vi "high_speed_digitizer_ao.vi"() -> ()   [LabVIEW 2014]
uses:
  <vilib>/Utility/error.llb/DialogType.ctl
  <vilib>/addons/h5labview2/file/H5Fmode.ctl
  <vilib>/DAQmx/create/channels.llb/DAQmx Create Channel (AI-Voltage-Basic).vi
  <vilib>/DAQmx/configure/timing.llb/DAQmx Timing (Sample Clock).vi
  <vilib>/DAQmx/create/channels.llb/DAQmx Create Channel (AO-Voltage-Basic).vi
  <vilib>/DAQmx/configure/trigger.llb/DAQmx Start Trigger (Digital Edge).vi
  <vilib>/DAQmx/configure/trigger.llb/DAQmx Start Trigger (Analog Edge).vi
  <vilib>/DAQmx/configure/trigger.llb/DAQmx Reference Trigger (Digital Edge).vi
  <vilib>/DAQmx/configure/trigger.llb/DAQmx Reference Trigger (Analog Edge).vi
  <vilib>/DAQmx/read.llb/DAQmx Read (Analog 2D DBL NChan NSamp).vi
  <vilib>/DAQmx/write.llb/DAQmx Write (Analog Wfm 1Chan NSamp).vi
  <vilib>/addons/h5labview2/base/lib_path.vi
  <vilib>/addons/h5labview2/base/H5Equery.vi
  <vilib>/addons/h5labview2/dataset/H5Dwrite.llb/H5Dwrite.xnode
  <vilib>/addons/h5labview2/attrib/H5Awrite.llb/H5Awrite.xnode
  <vilib>/addons/h5labview2/base/hid_t.ctl
  <resource>/objmgr/daqmx.rc
  <vilib>/addons/h5labview2/file/H5F.lvlib
  <vilib>/addons/h5labview2/group/H5G.lvlib
  National Instruments Downloads/LabVIEW FPGA English/FPGA Timekeeper 1.1b0/FPGA Timekeeper.lvlib
  <vilib>/measure/NI_MABase.lvlib
panel:
  in  "proc_amp_increment":dbl
  in  "proc_amp":dbl format="%0.2p"
  in  "synth_settle_time":u32
  in  "drive frequency increment":dbl
  in  "init drive frequency":dbl format="%0.2p"
  in  "drive amp increment":dbl
  in  "init drive amp":dbl format="%0.5p"
  in  "dc increment":dbl
  in  "init offset":dbl format="%0.2p"
  in  "Max Voltage 2":dbl=5.0
  in  "Min Voltage 2":dbl=-5.0
  in  "Physical Channel(s)":tag="Dev1/ao0"
  out "P_baratron [mbar]":dbl format="%#_3g"
  out "P_pirani [torr]":dbl format="%#_3g"
  out "P_cc [torr]":dbl format="%#_3g"
  out "T_elec_rack [C]":dbl
  out "T_opt_table [C]":dbl
  in  "Read pressures?":bool=TRUE
  in  "Read temps?":bool=TRUE
  in  "Num files":i32
  in  "File base name":string
  in  "Directory path":path
  out "Waveform Graph":dbl[][](graph)
  in  "Number of Samples":i32=500000
  in  "Trigger Type":T1(tab)=enum."Digital Start"
  in  "Edge":i32(ring)=10280 items=["Rising"=10280, "Falling"=10171]
  in  "Digital Trigger Source":tag="/Dev2/PFI0"
  in  "Level (V)":dbl format="%0.2f"
  in  "Hysteresis (V)":dbl
  in  "Slope":i32(ring)=10280 items=["Rising"=10280, "Falling"=10171]
  in  "Analog Trigger Source":string="APFI0"
  in  "Digital Ref Trigger Source":tag
  in  "Edge 2":i32(ring)=10280 items=["Rising"=10280, "Falling"=10171]
  in  "Pre-Trigger Samples":u32
  in  "Analog Ref Trigger Source":string="APFI0"
  in  "Slope 2":i32(ring)=10280 items=["Rising"=10280, "Falling"=10171]
  in  "Level (V) 2":dbl format="%0.2f"
  in  "Pre-Trigger Samples 2":u32
  in  "Sample Rate":dbl=300000.0
  in  "Sample Clock Source":tag="OnboardClock"
  in  "Terminal Configuration":i32(ring)=-1 items=["default"=-1, "RSE"=10083, "NRSE"=10078, "Differential"=10106, "Pseudodifferential"=12529]
  in  "Max Voltage":dbl=5.0
  in  "Min Voltage":dbl=-5.0
  in  "Physical Channel":tag="Dev2/ai0:2"
  out "Actual Sample Rate":dbl=1000.0 format="%0.2f"
  # "To configure and use a start trigger you must have the necessary tab selected above.  Not all hardware supports triggering--refer to your device documentation for more info."
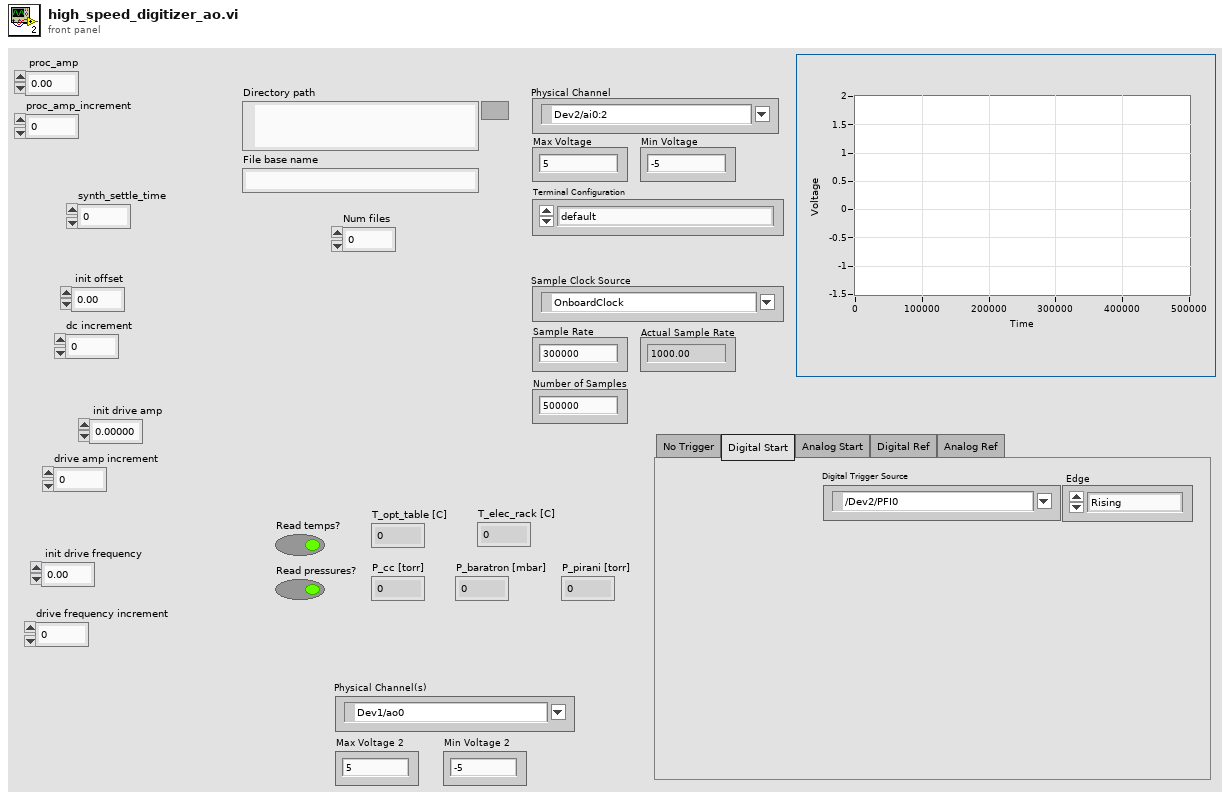
[diagram p1: front panel]
types:
  T1 = enum32{"No Trigger", "Digital Start", "Analog Start", "Digital Ref", "Analog Ref"}
  T2 = enum16{"Sine Wave", "Triangle Wave", "Square Wave", "Sawtooth Wave"}
  T3 = typedef "H5F.lvlib/H5Fmode.ctl" = enum16{"read-only", "read-write", "overwrite", "create new", "open or create"}
  T4 = typedef "DialogType.ctl" = u16
  T5 = typedef "hid_t.ctl" = i32
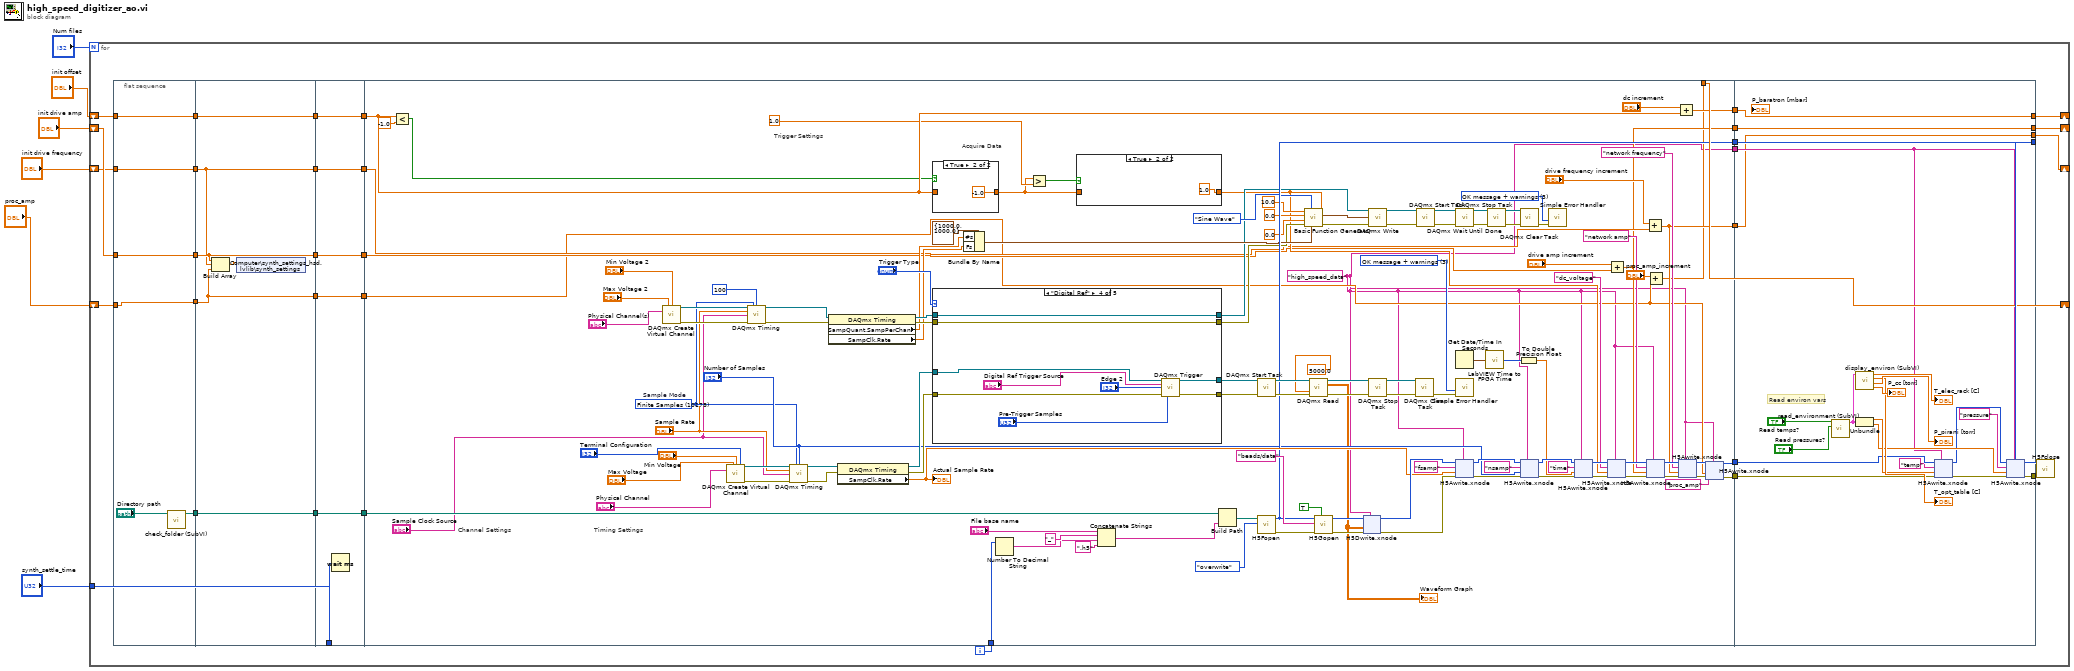
[diagram p0: block diagram]
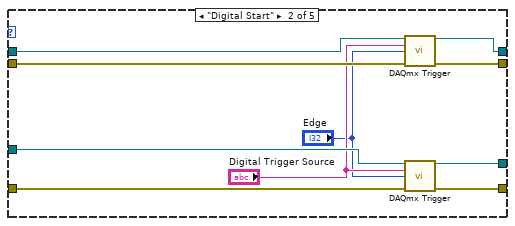
[diagram p5: hidden frame]
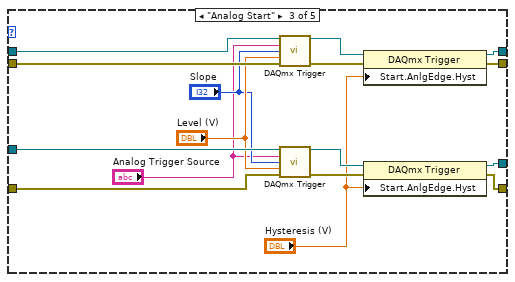
[diagram p6: hidden frame]
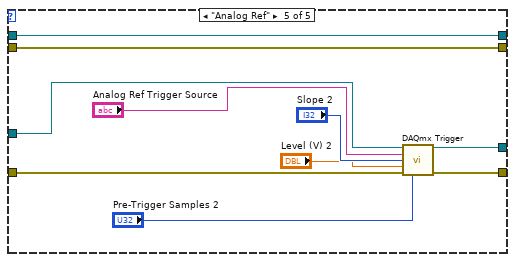
[diagram p7: hidden frame]
diagram:
  n1 = for {
    N: "Num files" -> [_]
    shift-right: [w32] -> _
    shift-left: "init offset" -> [w31]
    shift-right: [w20] -> _
    shift-left: "init drive amp" -> [w23]
    shift-right: [w13] -> _
    shift-left: "init drive frequency" -> [w18]
    tunnel: "synth_settle_time" -> [w12]
    shift-right: [w7] -> _
    shift-left: "proc_amp" -> [w10]
    i -> [w40]
    n2 = flat-sequence {
      tunnel: [w45] -> w30
      tunnel: [w44] -> w29
      tunnel: w31 -> [w44]
      tunnel: [w43] -> w24
      tunnel: w23 -> [w43]
      tunnel: w18 -> [w42]
      tunnel: [w42] -> w15
      tunnel: [w41] -> w11
      tunnel: w10 -> [w41]
      tunnel: w30 -> [w52]
      tunnel: [w52] -> w28
      tunnel: w29 -> [w51]
      tunnel: [w51] -> w26
      tunnel: w24 -> [w50]
      tunnel: [w50] -> w22
      tunnel: [w49] -> w16
      tunnel: w15 -> [w49]
      tunnel: w11 -> [w47]
      tunnel: [w47] -> w8
      tunnel: w28 -> [w58]
      tunnel: [w58] -> w27
      tunnel: w26 -> [w57]
      tunnel: [w57] -> w25
      tunnel: w22 -> [w56]
      tunnel: [w56] -> w21
      tunnel: [w55] -> w17
      tunnel: w16 -> [w55]
      tunnel: w12 -> [w54]
      tunnel: [w53] -> w9
      tunnel: w8 -> [w53]
      tunnel: w40 -> [w157]
      tunnel: [w137] -> w37
      tunnel: [w66] -> w36
      tunnel: [w64] -> w35
      tunnel: [w61] -> w34
      tunnel: w27 -> [w130]
      tunnel: w25 -> [w95]
      tunnel: [w92] -> w33
      tunnel: w21 -> [w80]
      tunnel: [w71] -> w19
      tunnel: w17 -> [w78]
      tunnel: [w70] -> w14
      tunnel: w9 -> [w63]
      tunnel: [w68] -> w7
      tunnel: [w386] -> w38
      tunnel: [w396] -> w39
      tunnel: w37 -> [w396]
      tunnel: w36 -> [w388]
      tunnel: w35 -> [w383]
      tunnel: w34 -> [w381]
      tunnel: [w378] -> w32
      tunnel: w33 -> [w378]
      tunnel: [w377] -> w20
      tunnel: w19 -> [w377]
      tunnel: [w376] -> w13
      tunnel: w14 -> [w376]
      frame #0 {
        n3 = call "check_folder (SubVI).vi"("path in"="Directory path") -> ("path out"=w45:path)  [unwired: 10 in]
      }
      frame #1 {
        n4 = Build Array(w50, w49, w47) -> (w48:dbl[])
        n5 = shared-variable "My Computer\\synth_settings_hsd.lvlib\\synth_settings"(w48) -> ()  [unwired: 1 in, 1 out]
      }
      frame #2 {
        n6 = Wait (ms)(milliseconds to wait=w54) -> ()  [unwired: 1 out]
      }
      frame #3 {
        w106 = T4 3 items=["no dialog", "OK message", "continue or stop message", "OK message + warnings", "continue/stop + warnings"] ("type of dialog (OK msg:1)")
        w61 = "high_speed_data" ("dataset name")
        w160 = T4 3 items=["no dialog", "OK message", "continue or stop message", "OK message + warnings", "continue/stop + warnings"] ("type of dialog (OK msg:1)")
        w99 = 10178 items=["Finite Samples"=10178, "Continuous Samples"=10123, "Hardware Timed Single Point"=12522]  # Sample Mode
        # "Acquire Data"
        # "Trigger Settings"
        # "Timing Settings"
        # "Channel Settings"
        n7 = Less?(x=w95, y=-1.0) -> (x < y?=w93:bool)
        n8 = call-poly <vilib>:"DAQmx Create Virtual Channel.vi"("maximum value"="Max Voltage 2", "minimum value"="Min Voltage 2", "physical channels"="Physical Channel(s)") -> ("task out"=w126:refnum<k21>, "error out"=w127:errorcluster)  [unwired: 11 in]
        n9 = call-poly <vilib>:"DAQmx Create Virtual Channel.vi"("maximum value"="Max Voltage", "minimum value"="Min Voltage", "input terminal configuration"="Terminal Configuration", "physical channels"="Physical Channel") -> ("task out"=w175:refnum<k21>, "error out"=w176:errorcluster)  [unwired: 10 in]
        n10 = call-poly <vilib>:"DAQmx Timing.vi"("task/channels in"=w126, "sample mode"=w99, "samples per channel"=100, "rate"="Sample Rate", "source"="Sample Clock Source", "error in"=w127) -> ("task out"=w129:refnum<k21>, "error out"=w128:errorcluster)  [unwired: 8 in]
        n11 = call-poly <vilib>:"DAQmx Timing.vi"("task/channels in"=w175, "sample mode"=w99, "samples per channel"="Number of Samples", "rate"="Sample Rate", "source"="Sample Clock Source", "error in"=w176) -> ("task out"=w178:refnum<k21>, "error out"=w177:errorcluster)  [unwired: 8 in]
        n12 = property class="DAQmx Timing"(reference=w129, error in=w128) -> (reference out=w122:refnum<k21>, error out=w121:errorcluster, "SampQuant.SampPerChan"=w119:dbl, "SampClk.Rate"=w118:dbl)
        n13 = property class="DAQmx Timing"(reference=w178, error in=w177) -> (reference out=w158:refnum<k21>, error out=w159:errorcluster, "SampClk.Rate"=w139:dbl)
        "Actual Sample Rate" <- w139
        n14 = case shown="True" w93 {
          tunnel: w95 -> [w235 _]
          tunnel: [w235 -1.0 ("offset")] -> w89
          frame False {
          }
          frame True {
          }
        }
        n15 = case shown="\"Digital Ref\"" "Trigger Type" {
          tunnel: w158 -> [w330 w340 w356 w365 w375]
          tunnel: w159 -> [w329 w339 w355 w364 w374]
          tunnel: [w330 w338 w354 w363 w369] -> w174
          tunnel: [w329 w337 w353 w362 w370] -> w173
          tunnel: w122 -> [w328 w336 w348 w358 w367]
          tunnel: w121 -> [w327 w335 w347 w357 w366]
          tunnel: [w328 w334 w346 w358 w367] -> w111
          tunnel: [w327 w333 w345 w357 w366] -> w113
          frame "No Trigger", Default {
          }
          frame "Digital Start" {
            n16 = call-poly <vilib>:"DAQmx Trigger.vi"("task/channels in"=w336, "source"="Digital Trigger Source", "edge"="Edge", "error in"=w335) -> ("task out"=w334:refnum<k21>, "error out"=w333:errorcluster)  [unwired: 10 in]
            n17 = call-poly <vilib>:"DAQmx Trigger.vi"("task/channels in"=w340, "source"="Digital Trigger Source", "edge"="Edge", "error in"=w339) -> ("task out"=w338:refnum<k21>, "error out"=w337:errorcluster)  [unwired: 10 in]
          }
          frame "Analog Start" {
            n18 = call-poly <vilib>:"DAQmx Trigger.vi"("task/channels in"=w348, "source"="Analog Trigger Source", "slope"="Slope", "level"="Level (V)", "error in"=w347) -> ("task out"=w350:refnum<k21>, "error out"=w349:errorcluster)  [unwired: 9 in]
            n19 = call-poly <vilib>:"DAQmx Trigger.vi"("task/channels in"=w356, "source"="Analog Trigger Source", "slope"="Slope", "level"="Level (V)", "error in"=w355) -> ("task out"=w352:refnum<k21>, "error out"=w351:errorcluster)  [unwired: 9 in]
            n20 = property class="DAQmx Trigger"(reference=w350, error in=w349, "Start.AnlgEdge.Hyst"="Hysteresis (V)") -> (reference out=w346:refnum<k21>, error out=w345:errorcluster)
            n21 = property class="DAQmx Trigger"(reference=w352, error in=w351, "Start.AnlgEdge.Hyst"="Hysteresis (V)") -> (reference out=w354:refnum<k21>, error out=w353:errorcluster)
          }
          frame "Digital Ref" {
            n22 = call-poly <vilib>:"DAQmx Trigger.vi"("task/channels in"=w365, "source"="Digital Ref Trigger Source", "edge"="Edge 2", "error in"=w364, "pretrigger samples per channel"="Pre-Trigger Samples") -> ("task out"=w363:refnum<k21>, "error out"=w362:errorcluster)  [unwired: 9 in]
          }
          frame "Analog Ref" {
            n23 = call-poly <vilib>:"DAQmx Trigger.vi"("task/channels in"=w375, "source"="Analog Ref Trigger Source", "slope"="Slope 2", "level"="Level (V) 2", "error in"=w374, "pretrigger samples per channel"="Pre-Trigger Samples 2") -> ("task out"=w369:refnum<k21>, "error out"=w370:errorcluster)  [unwired: 8 in]
          }
        }
        n24 = Bundle By Name(cluster=cluster{"Fs":dbl, "#s":dbl} {"Fs"=1000.0, "#s"=1000.0} ("sampling info"), "#s"=w119, "Fs"=w118) -> (w117:cluster{"Fs":dbl, "#s":dbl})
        n25 = Number To Decimal String(number=w157) -> (decimal integer string=w155:string)  [unwired: 1 in]
        n26 = Greater?(x=w89, y=1.0) -> (0:w90:bool)
        n27 = case shown="True" w90 {
          tunnel: w89 -> [w233 _]
          tunnel: [w233 1.0 ("offset")] -> w87
          frame False {
          }
          frame True {
          }
        }
        n28 = Concatenate Strings("File base name", "_", w155, ".h5") -> (w152:string)
        n29 = Build Path(base path=w130, name or relative path=w152) -> (appended path=w150:path)
        n30 = call <vilib>:"DAQmx Start Task.vi"("task/channels in"=w174, "error in"=w173) -> ("task out"=w172:refnum<k21>, "error out"=w171:errorcluster)  [unwired: 12 in]
        n31 = call <vilib>:"H5Fopen.vi"("mode (read-only)"=H5Fmode."overwrite", "path"=w150) -> ("error out"=w148:errorcluster, "ref out"=w137:T5)  [unwired: 8 in]
        n32 = call <vilib>:"Basic Function Generator.vi"("offset"=w87, "sampling info"=w117, "signal type"=T2."Sine Wave", "error in (no error)"=w113, "phase"=0.0, "amplitude"=0.0, "frequency"=10.0) -> ("error out"=w110:errorcluster, "signal out"=w86:waveform(dbl))  [unwired: 2 in, 1 out]
        n33 = call-poly <vilib>:"DAQmx Read.vi"("task/channels in"=w172, "timeout"=5000.0, "error in"=w171) -> ("task out"=w162:refnum<k21>, "data"=w60:dbl[][], "error out"=w161:errorcluster)  [unwired: 10 in]
        "Waveform Graph" <- w60
        n34 = call <vilib>:"H5Gopen.vi"("create? (F)"=TRUE, "error in (no error)"=w148, "name"="beads/data", "ref in"=w137) -> ("error out"=w147:errorcluster, "group out"=w146:T5)  [unwired: 6 in]
        n35 = xnode "H5Dwrite.xnode"("dataset name"=w61, "error in (no error)"=w147, "data"=w60, "ref in"=w146) -> ("error out"=w144:errorcluster, "ref out"=w145:i32)  [unwired: 3 in, 1 out]
        n36 = call-poly <vilib>:"DAQmx Write.vi"("task/channels in"=w111, "data"=w86, "error in"=w110) -> ("task out"=w105:refnum<k21>, "error out"=w104:errorcluster)  [unwired: 10 in, 1 out]
        n37 = call <vilib>:"DAQmx Stop Task.vi"("task/channels in"=w162, "error in"=w161) -> ("task out"=w164:refnum<k21>, "error out"=w163:errorcluster)  [unwired: 12 in]
        n38 = call <vilib>:"DAQmx Clear Task.vi"("task in"=w164, "error in"=w163) -> ("error out"=w170:errorcluster)  [unwired: 13 in]
        n39 = call <vilib>:"DAQmx Start Task.vi"("task/channels in"=w105, "error in"=w104) -> ("task out"=w85:refnum<k21>, "error out"=w83:errorcluster)  [unwired: 12 in]
        n40 = call <vilib>:"DAQmx Wait Until Done.vi"("task/channels in"=w85, "error in"=w83) -> ("task out"=w84:refnum<k21>, "error out"=w82:errorcluster)  [unwired: 12 in]
        n41 = Get Date/Time In Seconds() -> (seconds since 1Jan1904=w133:timestamp)
        n42 = call <vilib>:"Simple Error Handler.vi"("type of dialog (OK msg:1)"=w160, "error in (no error)"=w170) -> ()  [unwired: 3 in, 5 out]
        n43 = xnode "H5Awrite.xnode"("object name"=w61, "error in (no error)"=w144, "data"=w139, "attrib name"="fsamp", "ref in"=w145) -> ("error out"=w142:errorcluster, "ref out"=w143:T5)  [unwired: 2 in, 1 out]
        n44 = call "LabVIEW Time to FPGA Time.vi"("LabVIEW time"=w133) -> ("FPGA time (ns)"=w132:u64)
        n45 = call <vilib>:"DAQmx Stop Task.vi"("task/channels in"=w84, "error in"=w82) -> ("task out"=w108:refnum<k21>, "error out"=w107:errorcluster)  [unwired: 12 in]
        n46 = call <vilib>:"DAQmx Clear Task.vi"("task in"=w108, "error in"=w107) -> ("error out"=w109:errorcluster)  [unwired: 13 in]
        n47 = To Double Precision Float(number=w132) -> (double precision float=w131:dbl)
        n48 = xnode "H5Awrite.xnode"("object name"=w61, "error in (no error)"=w142, "data"="Number of Samples", "attrib name"="nsamp", "ref in"=w143) -> ("error out"=w135:errorcluster, "ref out"=w136:T5)  [unwired: 2 in, 1 out]
        n49 = call <vilib>:"Simple Error Handler.vi"("type of dialog (OK msg:1)"=w106, "error in (no error)"=w109) -> ()  [unwired: 3 in, 5 out]
        n50 = xnode "H5Awrite.xnode"("object name"=w61, "error in (no error)"=w135, "data"=w131, "attrib name"="time", "ref in"=w136) -> ("error out"=w103:errorcluster, "ref out"=w102:T5)  [unwired: 2 in, 1 out]
        n51 = xnode "H5Awrite.xnode"("object name"=w61, "error in (no error)"=w103, "data"=w87, "attrib name"="dc_voltage", "ref in"=w102) -> ("error out"=w77:errorcluster, "ref out"=w75:T5)  [unwired: 2 in, 1 out]
        n52 = Add(x="drive amp increment", y=w80) -> (x+y=w71:dbl)
        n53 = Add(x="drive frequency increment", y=w78) -> (x+y=w70:dbl)
        n54 = xnode "H5Awrite.xnode"("object name"=w61, "error in (no error)"=w77, "data"=w71, "attrib name"="network amp", "ref in"=w75) -> ("error out"=w76:errorcluster, "ref out"=w74:T5)  [unwired: 2 in, 1 out]
        n55 = Add(x="proc_amp_increment", y=w63) -> (x+y=w68:dbl)
        n56 = Add(x="dc increment", y=w95) -> (x+y=w92:dbl)
        n57 = xnode "H5Awrite.xnode"("object name"=w61, "error in (no error)"=w76, "data"=w70, "attrib name"="network frequency", "ref in"=w74) -> ("error out"=w67:errorcluster, "ref out"=w65:T5)  [unwired: 2 in, 1 out]
        n58 = xnode "H5Awrite.xnode"("object name"=w61, "error in (no error)"=w67, "data"=w63, "attrib name"="proc_amp", "ref in"=w65) -> ("error out"=w66:errorcluster, "ref out"=w64:T5)  [unwired: 2 in, 1 out]
      }
      frame #4 {
        # "Read environ vars"
        n59 = call "read_environment (SubVI).vi"("Read pressures?"="Read pressures?", "Read temps?"="Read temps?") -> ("environ cluster"=w389:cluster{dbl[], dbl[]})  [unwired: 9 in]
        n60 = call "display_environ (SubVI).vi"("environ cluster"=w389) -> ("P_pirani"=→"P_cc [torr]":dbl, "P_cc"=→"P_pirani [torr]":dbl, "T_opt_table"=→"T_opt_table [C]":dbl, "T_elec_rack"=→"T_elec_rack [C]":dbl)  [unwired: 6 in, 1 out]
        n61 = Unbundle(w389) -> (w385:dbl[], w384:dbl[])
        n62 = xnode "H5Awrite.xnode"("object name"=w381, "error in (no error)"=w388, "data"=w385, "attrib name"="temp", "ref in"=w383) -> ("error out"=w387:errorcluster, "ref out"=w382:T5)  [unwired: 2 in, 1 out]
        n63 = xnode "H5Awrite.xnode"("object name"=w381, "error in (no error)"=w387, "data"=w384, "attrib name"="pressure", "ref in"=w382) -> ("error out"=w386:errorcluster)  [unwired: 2 in, 2 out]
      }
    }
    n64 = call <vilib>:"H5Fclose.vi"("error in (no error)"=w38, "ref"=w39) -> ()  [unwired: 9 in, 1 out]
  }
